vi "05.1-2 Managing Initialization Files (.ini).vi"() -> ()   [LabVIEW 2019]
uses:
  <vilib>/Utility/config.llb/Write Key (Double).vi
  <vilib>/Utility/config.llb/Read Key (Double).vi
  <vilib>/Utility/config.llb/NI_LVConfig.lvlib
panel:
  out "found?":bool
  out "value":dbl
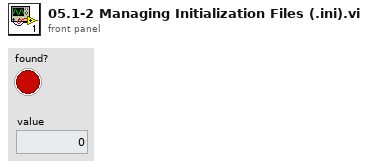
[diagram p1: front panel]
types:
  T1 = enum16{"fractional", "engineering", "exponential"}
  T2 = typedef "NI_LVConfig.lvlib/Config Data RefNum.ctl" = refnum<k1>
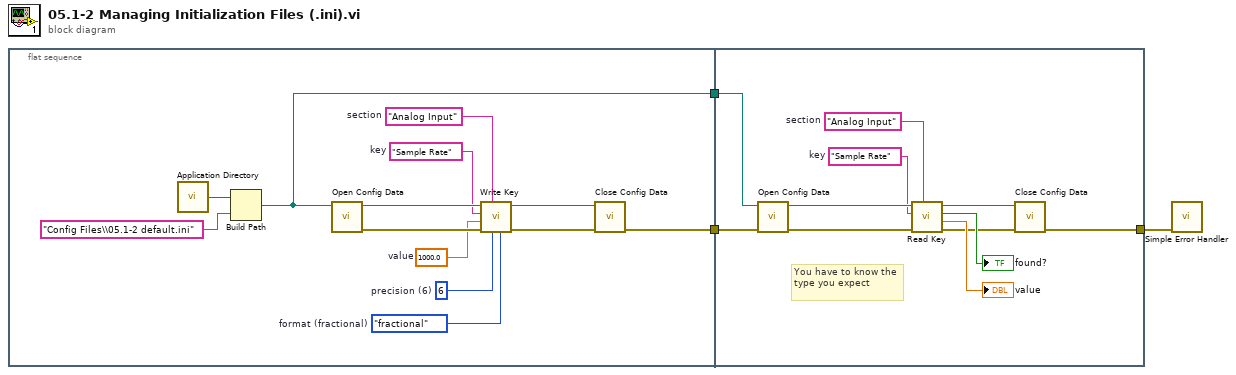
[diagram p0: block diagram]
diagram:
  n1 = flat-sequence {
    tunnel: [w5] -> w3
    tunnel: [w4] -> w2
    tunnel: w3 -> [w26]
    tunnel: w2 -> [w27]
    tunnel: [w17] -> w1
    frame #0 {
      w6 = T1."fractional"  # format (fractional)
      w7 = i16 6  # precision (6)
      w8 = 1000.0  # value
      w11 = "Sample Rate"  # key
      w12 = "Analog Input"  # section
      n2 = call <vilib>:"Application Directory.vi"() -> ("Application Directory"=w16:path)
      n3 = Build Path(base path=w16, name or relative path="Config Files\\05.1-2 default.ini") -> (appended path=w5:path)
      n4 = call <vilib>:"Open Config Data.vi"("configuration file path"=w5) -> ("error out"=w13:errorcluster, "refnum"=w14:T2)  [unwired: 8 in, 1 out]
      n5 = call-poly <vilib>:"Write Key.vi"("format (fractional)"=w6, "precision (6)"=w7, "section"=w12, "error in (no error)"=w13, "value"=w8, "key"=w11, "refnum"=w14) -> ("error out"=w9:errorcluster, "refnum out"=w10:T2)  [unwired: 2 in, 1 out]
      n6 = call <vilib>:"Close Config Data.vi"("error in (no error)"=w9, "refnum"=w10) -> ("error out"=w4:errorcluster)  [unwired: 8 in, 1 out]
    }
    frame #1 {
      w23 = "Sample Rate"  # key
      w22 = "Analog Input"  # section
      # "You have to know the type you expect"
      n7 = call <vilib>:"Open Config Data.vi"("error in (no error)"=w27, "configuration file path"=w26) -> ("error out"=w24:errorcluster, "refnum"=w25:T2)  [unwired: 7 in, 1 out]
      n8 = call-poly <vilib>:"Read Key.vi"("section"=w22, "error in (no error)"=w24, "key"=w23, "refnum"=w25) -> ("error out"=w19:errorcluster, "value"=→"value":dbl, "found?"=→"found?":bool, "refnum out"=w18:T2)  [unwired: 4 in]
      n9 = call <vilib>:"Close Config Data.vi"("error in (no error)"=w19, "refnum"=w18) -> ("error out"=w17:errorcluster)  [unwired: 8 in, 1 out]
    }
  }
  n10 = call <vilib>:"Simple Error Handler.vi"("error in (no error)"=w1) -> ()  [unwired: 4 in, 5 out]
